vi "Run Tests with Simulated Devices.vi"() -> ()   [LabVIEW 2023]
uses:
  <vilib>/addons/_JKI Toolkits/Caraya/classes/Assert/Assert Not Error.vi
panel:
  out "error out":errorcluster
  in  "error in (no error)":errorcluster
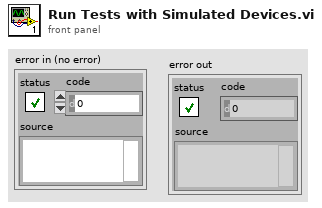
[diagram p1: front panel]
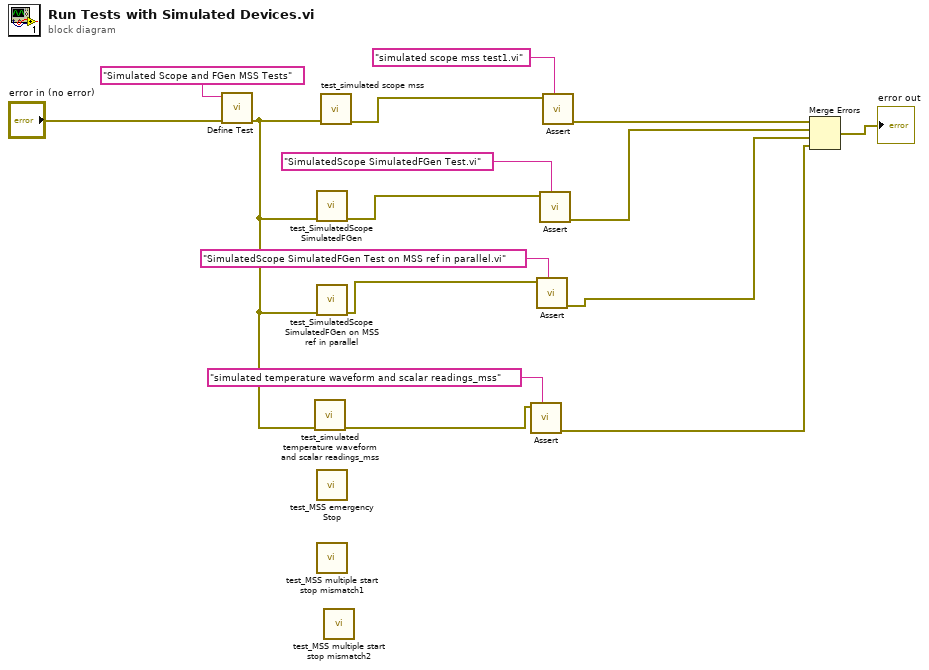
[diagram p0: block diagram]
diagram:
  n1 = call <vilib>:"Define Test.vi"("error in (no error)"="error in (no error)", "Label (VI Title)"="Simulated Scope and FGen MSS Tests") -> ("error out"=w2:errorcluster)  [unwired: 8 in, 1 out]
  n2 = call "test_simulated temperature waveform and scalar readings_mss.vi"("Error In"=w2) -> ("Error Out"=w3:errorcluster)  [unwired: 10 in]
  n3 = call "test_SimulatedScope SimulatedFGen.vi"("Error In"=w2) -> ("Error Out"=w13:errorcluster)  [unwired: 10 in]
  n4 = call "test_SimulatedScope SimulatedFGen on MSS ref in parallel.vi"("Error In"=w2) -> ("Error Out"=w5:errorcluster)  [unwired: 10 in]
  n5 = call "test_MSS emergency Stop.vi"() -> ()  [unwired: 11 in, 1 out]
  n6 = call "test_MSS multiple start stop mismatch1.vi"() -> ()  [unwired: 11 in, 1 out]
  n7 = call "test_simulated scope mss.vi"("Error In"=w2) -> ("Error Out"=w15:errorcluster)  [unwired: 10 in]
  n8 = call "test_MSS multiple start stop mismatch2.vi"() -> ()  [unwired: 11 in, 1 out]
  n9 = call-poly <vilib>:"Assert.vi"("Label"="simulated temperature waveform and scalar readings_mss", "Not Error?"=w3) -> ("error out"=w1:errorcluster)  [unwired: 8 in, 1 out]
  n10 = call-poly <vilib>:"Assert.vi"("Label"="SimulatedScope SimulatedFGen Test on MSS ref in parallel.vi", "Not Error?"=w5) -> ("error out"=w6:errorcluster)  [unwired: 8 in, 1 out]
  n11 = call-poly <vilib>:"Assert.vi"("Label"="SimulatedScope SimulatedFGen Test.vi", "Not Error?"=w13) -> ("error out"=w11:errorcluster)  [unwired: 8 in, 1 out]
  n12 = call-poly <vilib>:"Assert.vi"("Label"="simulated scope mss test1.vi", "Not Error?"=w15) -> ("error out"=w16:errorcluster)  [unwired: 8 in, 1 out]
  n13 = Merge Errors(w16, w11, w6, w1) -> (→"error out":errorcluster)
